vi "Default Buffer Converter Name.vi"() -> (2 "component name":string)   [LabVIEW 2020, in "DSF Configuration API.lvlib"]
uses:
  DSF Configuration API.lvlib
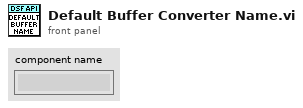
[diagram p1: front panel]
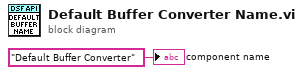
[diagram p0: block diagram]
diagram:
  "component name" <- "Default Buffer Converter" ("component name")
